vi "PH_Tektronix_7000.Evt Call Init.vi"(0 "i ref in":refnum<vi>, 1 "Instance":string="N/A", 5 "error in (no error)":errorcluster) -> (14 "i ref out":refnum<vi>, 19 "error out":errorcluster)   [LabVIEW 2014, in "PH_Tektronix_7000.lvlib"]
doc: "This VI calls sets a simple call."
uses:
  PH_Tektronix_7000.lvlib
  CS_Core/BaseProcess/BaseProcess.lvlib
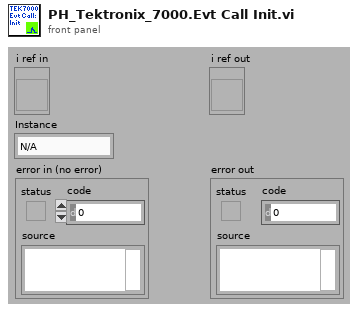
[diagram p1: front panel]
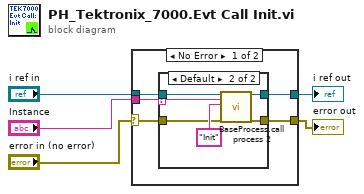
[diagram p0: block diagram]
diagram:
  n1 = case shown="No Error" "error in (no error)" {
    selector: "error in (no error)" -> [w6 w19]
    tunnel: [w10 w20] -> w5
    tunnel: [w9 w19] -> w4
    tunnel: "i ref in" -> [w8 w20]
    tunnel: "Instance" -> [w7 _]
    frame No Error {
      n2 = case shown="Default" w7 {
        selector: w7 -> [_ w13]
        tunnel: [w11 w17] -> w10
        tunnel: [w12 w16] -> w9
        tunnel: w8 -> [w11 w15]
        tunnel: w6 -> [w12 w14]
        frame "N/A" {
        }
        frame Default {
          n3 = call "BaseProcess.call process 2.vi"("i ref in"=w15, "Object"=w13, "Selector"="Init", "error in (no error)"=w14) -> ("i ref out"=w17:refnum<vi>, "error out"=w16:errorcluster)  [unwired: 14 in]
        }
      }
    }
    frame Error {
    }
  }
  "i ref out" <- w5
  "error out" <- w4
